vi "Get Channel FIFO locations.vi"(7 "Error On Missing Section? (T)":bool, 8 "error in (no error)":errorcluster, 9 "Channels to get refs":T2[](array[typedef]), 10 "Section By Relative Path (\"\")":string, 11 "Device Ref in":T1 format="%.0x") -> (0 "error out":errorcluster, 2 "FIFO Locations":i32[](array[numeric]), 3 "Device Ref out":T1 format="%.0x")   [LabVIEW 2015, in "NI Synchronization System Explorer.lvlib"]
uses:
  NI Synchronization System Explorer.lvlib
  Shared/Channel.ctl
  <vilib>/NI Veristand/Custom Device API/Custom Device Item Ref.ctl
  <vilib>/NI Veristand/Custom Device API/Custom Device API.lvlib
  <vilib>/NI Veristand/Custom Device Tools/Custom Device Utility Library/Custom Device Utility Library.lvlib
  Shared/NI Synchronization Shared.lvlib
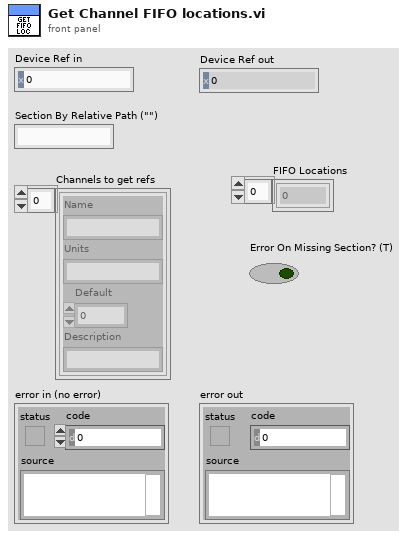
[diagram p1: front panel]
types:
  T1 = typedef "Custom Device API.lvlib/Custom Device Item Ref.ctl" = u64
  T2 = typedef "NI Synchronization Shared.lvlib/Channel.ctl" = cluster{"Name":string, "Units":string, "Default":dbl, "Description":string}
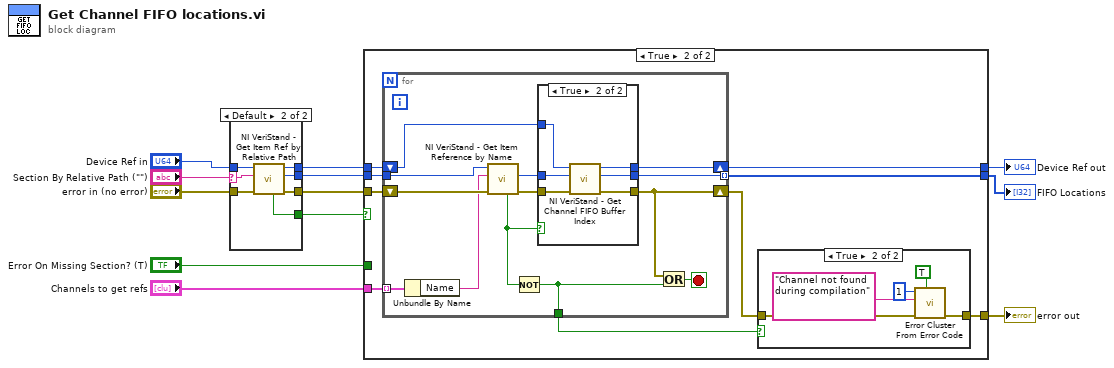
[diagram p0: block diagram]
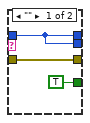
[diagram p2: hidden frame]
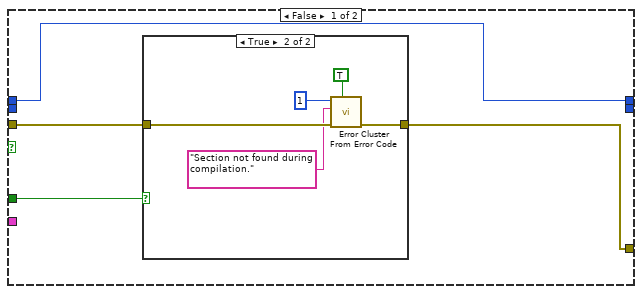
[diagram p3: hidden frame]
diagram:
  n1 = case shown="Default" "Section By Relative Path (\"\")" {
    selector: "Section By Relative Path (\"\")" -> [_ w16]
    tunnel: [w15 w22] -> w8
    tunnel: [w15 w21] -> w7
    tunnel: [w14 w20] -> w6
    tunnel: "Device Ref in" -> [w15 w19]
    tunnel: "error in (no error)" -> [w14 w18]
    tunnel: [TRUE ("Found") w17] -> w3
    frame "" {
    }
    frame Default {
      n2 = call <vilib>:"NI VeriStand - Get Item Ref by Relative Path.vi"("error in"=w18, "Relative Item Path"=w16, "Section Ref in"=w19) -> ("error out"=w20:errorcluster, "Item Ref"=w21:T1, "Section Ref out"=w22:T1, "Found"=w17:bool)  [unwired: 5 in]
    }
  }
  n3 = case shown="True" w3 {
    tunnel: [_ w41] -> w12
    tunnel: "Channels to get refs" -> [_ w40]
    tunnel: [w25 w39] -> w10
    tunnel: [w24 w33] -> w9
    tunnel: w8 -> [w25 w38]
    tunnel: w7 -> [_ w37]
    tunnel: w6 -> [w26 w36]
    tunnel: "Error On Missing Section? (T)" -> [w23 _]
    frame False {
      n4 = case shown="True" w23 {
        tunnel: w26 -> [w27 w32]
        tunnel: [w27 w31] -> w24
        frame False {
        }
        frame True {
          n5 = call <vilib>:"Error Cluster From Error Code.vi"("show call chain? (False)"=TRUE, "error in (no error)"=w32, "error message (\"\")"="Section not found during compilation." ("error message (\"\")"), "error code (0)"=1) -> ("error out"=w31:errorcluster)  [unwired: 5 in]
        }
      }
    }
    frame True {
      n6 = for {
        shift-right: [w54] -> w34
        shift-left: w36 -> [w60]
        tunnel: w37 -> [w59]
        tunnel: w40 -> [w58] mode=indexing
        tunnel: [w51] -> w41 mode=indexing
        shift-right: [w52] -> w39
        shift-left: w38 -> [w53]
        tunnel: [w55] -> w35
        stop <- w56 stop-if-true
        n7 = Unbundle By Name(w58) -> ("Name"=w48:string)
        n8 = call <vilib>:"NI VeriStand - Get Item Reference by Name.vi"("error in (no error)"=w60, "Item Name"=w48, "Parent Ref in"=w59) -> ("error out"=w57:errorcluster, "Item Ref"=w50:T1, "Found"=w49:bool)  [unwired: 5 in, 1 out]
        n9 = Not(x=w49) -> (.not. x?=w55:bool)
        n10 = case shown="True" w49 {
          tunnel: w57 -> [w61 w64]
          tunnel: [w61 w68] -> w54
          tunnel: w53 -> [w62 w67]
          tunnel: [w62 w66] -> w52
          tunnel: [_ w65] -> w51
          tunnel: w50 -> [_ w63]
          frame False {
          }
          frame True {
            n11 = call <vilib>:"NI VeriStand - Get Channel FIFO Buffer Index.vi"("error in"=w64, "Channel Ref"=w63, "Device Ref in"=w67) -> ("error out"=w68:errorcluster, "Channel FIFO Buffer Index"=w65:i32, "Device Ref out"=w66:T1)  [unwired: 4 in, 2 out]
          }
        }
        n12 = Or(x=w54, y=w55) -> (x .or. y?=w56:bool)
      }
      n13 = case shown="True" w35 {
        tunnel: w34 -> [w42 w47]
        tunnel: [w42 w46] -> w33
        frame False {
        }
        frame True {
          n14 = call <vilib>:"Error Cluster From Error Code.vi"("show call chain? (False)"=TRUE, "error in (no error)"=w47, "error message (\"\")"="Channel not found during compilation" ("error message (\"\")"), "error code (0)"=1) -> ("error out"=w46:errorcluster)  [unwired: 5 in]
        }
      }
    }
  }
  "Device Ref out" <- w10
  "error out" <- w9
  "FIFO Locations" <- w12
